vi "Export - Rx Packets.vi"(8 "error in (no error)":errorcluster, 11 "Device Item Ref in":T11 format="%.0x") -> (0 "error out":errorcluster, 3 "Rx Packets":T1 {"Rx Packet Data"."targetPriority" min=-2 max=16 step=1; "Rx Packet Data"."targetProcessor" min=-2 max=16 step=1; "Rx Packet Data"."Endianness" items=["big-endian"=0, "little-endian"=2]})   [LabVIEW 2019, in "UDP-Custom-Device System Explorer.lvlib"]
uses:
  UDP-Custom-Device System Explorer.lvlib
  <vilib>/NI VeriStand/Custom Device API/Custom Device Item Ref.ctl
  Types/XML - New/ImpExp - Rx Packets Data.ctl
  <vilib>/NI VeriStand/Custom Device API/Custom Device Item Info.ctl
  Types/XML - New/ImpExp - Rx Packet Data.ctl
  Shared/Types/Shared - Channel Data Type.ctl
  Shared/Types/Shared - Buffered.PacketInfo.ctl
  Shared/Types/Shared - Pointer Encoding.ctl
  Shared/Types/Shared - Receive Buffer Options.ctl
  Shared/Types/Shared - Transmit Buffer Options.ctl
  Shared/Types/Shared - New Data Options.ctl
  Shared/Types/Shared - Thread Management.ctl
  Shared/Constants.vi
  <vilib>/NI VeriStand/Custom Device API/Custom Device API.lvlib
  Property Accessors/Shared Section Accessors.lvlib
  Shared/UDP-Custom-Device Shared.lvlib
  Property Accessors/Shared Packet Accessors.lvlib
  <vilib>/NI VeriStand/Custom Device Tools/Custom Device Utility Library/Custom Device Utility Library.lvlib
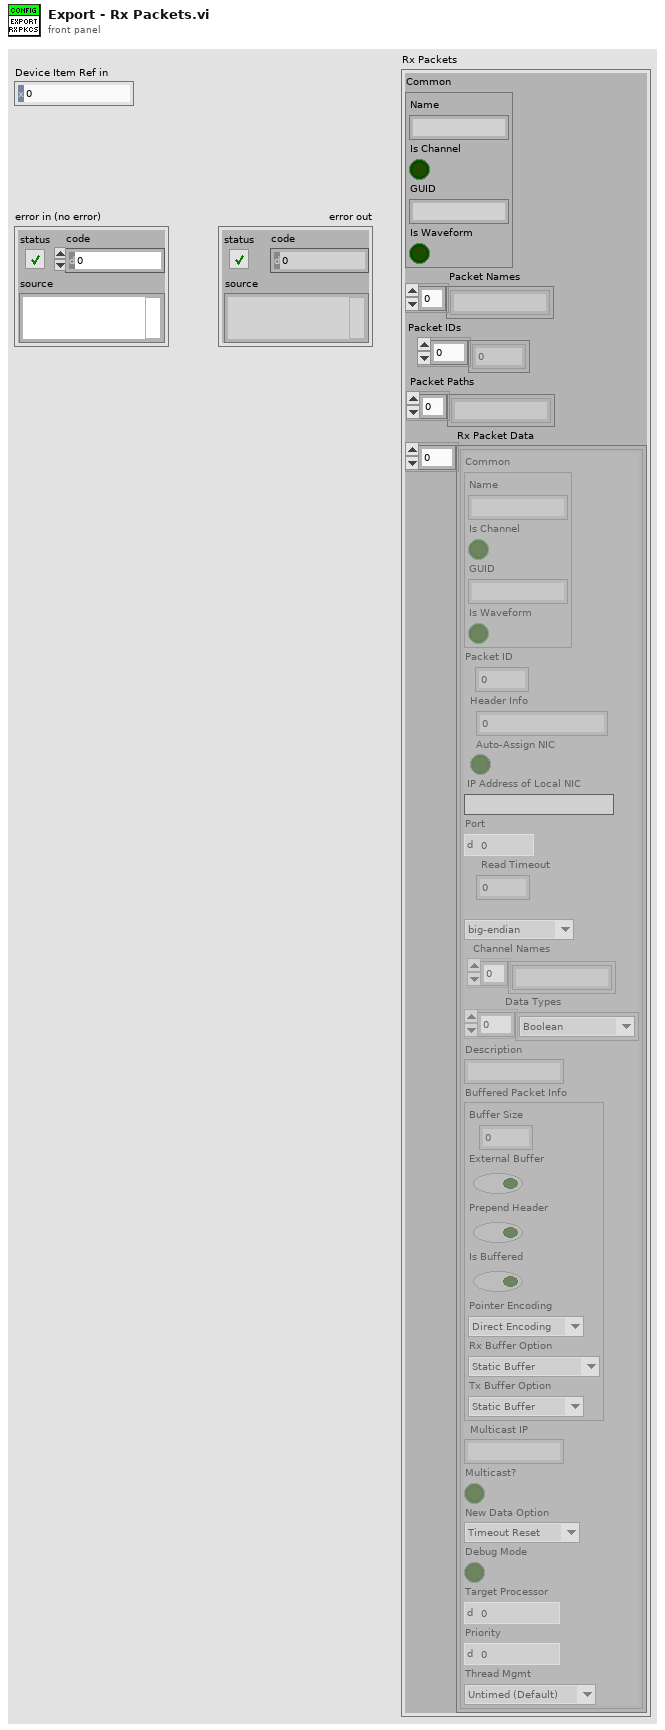
[diagram p1: front panel]
types:
  T1 = typedef "UDP-Custom-Device System Explorer.lvlib/ImpExp - Rx Packets Data.ctl" = cluster{"Common":T2, "Packet Names":string[], "Packet IDs":i32[], "Packet Paths":string[], "Rx Packet Data":T3[]}
  T2 = typedef "Custom Device API.lvlib/Custom Device Item Info.ctl" = cluster{"Name":string, "Is Channel":bool, "GUID":string, "Is Waveform":bool}
  T3 = typedef "UDP-Custom-Device System Explorer.lvlib/ImpExp - Rx Packet Data.ctl" = cluster{"Common":T2, "Packet ID":i32, "Header Info":u32, "Auto-Assign NIC":bool, "IP Address of Local NIC":string, "Port":u16, "Read Timeout":i32, "Endianness":u16, "Channel Names":string[], "Data Types":T4[], "Description":string, "Buffered Packet Info":T5, "Multicast IP":string, "Multicast?":bool, "New Data Option":T9, "Debug Mode":bool, "targetProcessor":i8, "targetPriority":i16, "Thread Mgmt":T10}
  T4 = typedef "UDP-Custom-Device Shared.lvlib/Shared - Channel Data Type.ctl" = enum16{"Boolean", "Single", "Double", "I8", "I16", "I32", "I64", "U8", "U16", "U32", "U64"}
  T5 = typedef "UDP-Custom-Device Shared.lvlib/Shared - Buffered.PacketInfo.ctl" = cluster{"Buffer Size":i32, "External Buffer":bool, "Prepend Header":bool, "Is Buffered":bool, "Pointer Encoding":T6, "Rx Buffer Option":T7, "Tx Buffer Option":T8}
  T6 = typedef "UDP-Custom-Device Shared.lvlib/Shared - Pointer Encoding.ctl" = enum16{"Direct Encoding", "Conversion Encoding"}
  T7 = typedef "UDP-Custom-Device Shared.lvlib/Shared - Receive Buffer Options.ctl" = enum16{"Static Buffer", "Circular Buffer", "Circular Buffer + Size", "Internal Cache", "Internal Cache + Size", "Ping Pong", "Ping Pong + Size"}
  T8 = typedef "UDP-Custom-Device Shared.lvlib/Shared - Transmit Buffer Options.ctl" = enum16{"Static Buffer", "FIFO Buffer", "FIFO Buffer + Port"}
  T9 = typedef "UDP-Custom-Device Shared.lvlib/Shared - New Data Options.ctl" = enum16{"Timeout Reset", "Counter"}
  T10 = typedef "UDP-Custom-Device Shared.lvlib/Shared - Thread Management.ctl" = enum16{"Untimed (Default)", "Timed (High Priority)"}
  T11 = typedef "Custom Device API.lvlib/Custom Device Item Ref.ctl" = u64
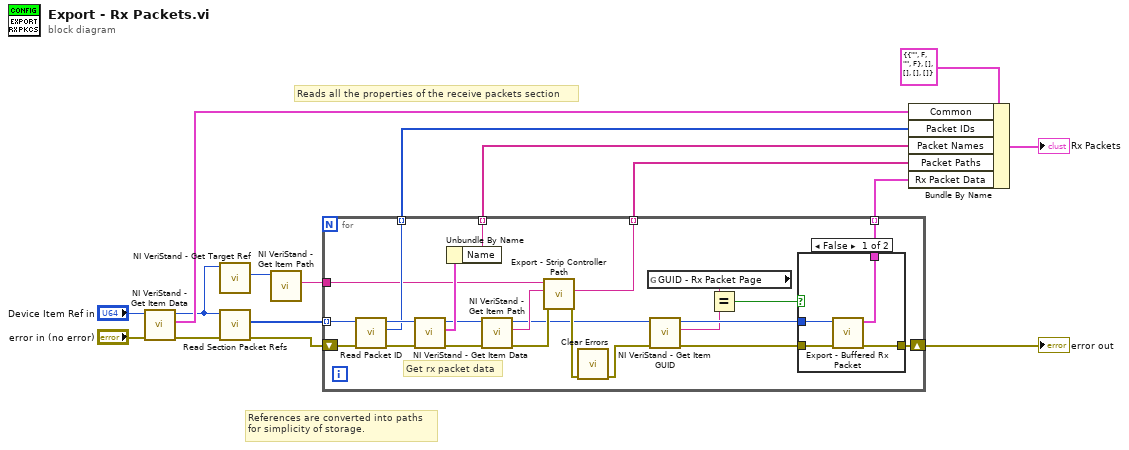
[diagram p0: block diagram]
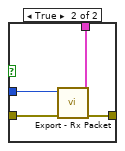
[diagram p2: hidden frame]
diagram:
  # "References are converted into paths\nfor simplicity of storage."
  # "Reads all the properties of the receive packets section"
  n1 = call <vilib>:"NI VeriStand - Get Item Data.vi"("error in (no error)"="error in (no error)", "Item Ref in"="Device Item Ref in") -> ("error out"=w6:errorcluster, "Item Info"=w10:T2, "Item Ref out"=w3:T11)  [unwired: 6 in, 1 out]
  n2 = call <vilib>:"NI VeriStand - Get Target Ref.vi"("Item Ref in"=w3) -> ("Target Ref"=w2:T11)  [unwired: 7 in, 3 out]
  n3 = call "Read Section Packet Refs.vi"("error in (no error)"=w6, "Node Ptr"=w3) -> ("error out"=w16:errorcluster, "Dependent Node Refs"=w15:T11[])  [unwired: 7 in, 1 out]
  n4 = call <vilib>:"NI VeriStand - Get Item Path.vi"("Item Ref in"=w2) -> ("Path"=w1:string)  [unwired: 7 in, 3 out]
  n5 = for {
    shift-right: [w39] -> w12
    shift-left: w16 -> [w33]
    tunnel: w15 -> [w31] mode=indexing
    tunnel: [w26] -> w9 mode=indexing
    tunnel: [w38] -> w7 mode=indexing
    tunnel: [w34] -> w5 mode=indexing
    tunnel: [w29] -> w4 mode=indexing
    tunnel: w1 -> [w28]
    # "Get rx packet data"
    n6 = call "Read Packet ID.vi"("error in (no error)"=w33, "Node Ptr"=w31) -> ("error out"=w32:errorcluster, "Packet ID"=w29:i32, "Node Ptr out"=w30:T11)  [unwired: 7 in]
    n7 = call <vilib>:"NI VeriStand - Get Item Data.vi"("error in (no error)"=w32, "Item Ref in"=w30) -> ("error out"=w35:errorcluster, "Item Info"=w37:T2, "Item Ref out"=w36:T11)  [unwired: 6 in, 1 out]
    n8 = Unbundle By Name(w37) -> ("Name"=w34:string)
    n9 = call <vilib>:"NI VeriStand - Get Item Path.vi"("error in (no error)"=w35, "Item Ref in"=w36) -> ("error out"=w25:errorcluster, "Path"=w27:string, "Item Ref out"=w23:T11)  [unwired: 6 in, 1 out]
    n10 = call "Export - Strip Controller Path.vi"("error in (no error)"=w25, "Channel Path"=w27, "Controller Path"=w28) -> ("error out"=w24:errorcluster, "Stripped Path"=w26:string)  [unwired: 7 in]
    n11 = call <vilib>:"Clear Errors.vi"("error in (no error)"=w24) -> ("error out"=w21:errorcluster)  [unwired: 5 in, 1 out]
    n12 = global read "Constants.vi" "GUID - Rx Packet Page"() -> (w19:string)
    n13 = call <vilib>:"NI VeriStand - Get Item GUID.vi"("error in (no error)"=w21, "Item Ref in"=w23) -> ("error out"=w20:errorcluster, "GUID"=w18:string, "Item Ref out"=w22:T11)  [unwired: 7 in]
    n14 = Equal?(x=w19, y=w18) -> (x = y?=w17:bool)
    n15 = case shown="False" w17 {
      tunnel: [w41 w47] -> w39
      tunnel: [w40 w46] -> w38
      tunnel: w22 -> [w43 w45]
      tunnel: w20 -> [w42 w44]
      frame False {
        n16 = call "Export - Buffered Rx Packet.vi"("error in (no error)"=w42, "Device Item Ref in"=w43) -> ("error out"=w41:errorcluster, "Rx Packet"=w40:T3)  [unwired: 8 in]
      }
      frame True {
        n17 = call "Export - Rx Packet.vi"("error in (no error)"=w44, "Device Item Ref in"=w45) -> ("error out"=w47:errorcluster, "Rx Packet"=w46:T3)  [unwired: 8 in]
      }
    }
  }
  "error out" <- w12
  n18 = Bundle By Name(cluster=T1 {"Common"={"Name"="", "Is Channel"=FALSE, "GUID"="", "Is Waveform"=FALSE}, "Packet Names"=[], "Packet IDs"=[], "Packet Paths"=[], "Rx Packet Data"=[]} ("Rx Packets"), "Common"=w10, "Packet IDs"=w4, "Packet Names"=w5, "Packet Paths"=w9, "Rx Packet Data"=w7) -> (→"Rx Packets":T1)
